vi "Open Help Topic.vi"(0 "Help file":string, 7 "HelpId":i32=-1, 11 "error in (no error)":errorcluster) -> (15 "error out":errorcluster)   [LabVIEW 2020]
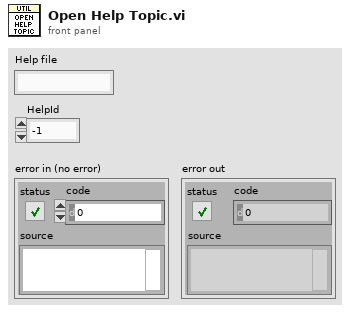
[diagram p1: front panel]
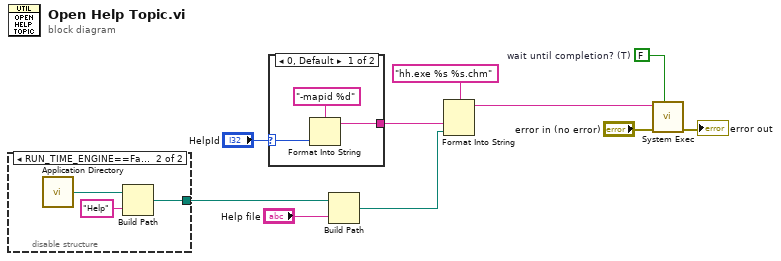
[diagram p0: block diagram]
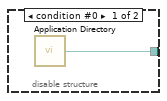
[diagram p2: hidden frame]
diagram:
  w10 = FALSE  # wait until completion? (T)
  n1 = disable-structure shown="RUN_TIME_ENGINE==False" {
    disable-tunnel: [w11 w13] -> w1
    frame condition #0 {
      n2 = call <vilib>:"Application Directory.vi"() -> ("Application Directory"=w11:path)
    }
    frame condition #1 (active) {
      n3 = call <vilib>:"Application Directory.vi"() -> ("Application Directory"=w14:path)
      n4 = Build Path(base path=w14, name or relative path="Help") -> (appended path=w13:path)
    }
  }
  n5 = case shown="0, Default" "HelpId" {
    selector: "HelpId" -> [w17 _]
    tunnel: [w15 _] -> w2
    frame 0, Default {
      n6 = Format Into String(format string="-mapid %d", w17) -> (resulting string=w15:string)  [unwired: 2 in, 1 out]
    }
    frame -1 {
    }
  }
  n7 = Build Path(base path=w1, name or relative path="Help file") -> (appended path=w5:path)
  n8 = Format Into String(format string="hh.exe %s %s.chm", w2, w5) -> (resulting string=w9:string)  [unwired: 2 in, 1 out]
  n9 = call <vilib>:"System Exec.vi"("wait until completion? (T)"=w10, "error in (no error)"="error in (no error)", "command line"=w9) -> ("error out"=→"error out":errorcluster)  [unwired: 5 in, 3 out]
